vi "Destroy.vi"(8 "error in (no error)":errorcluster, 11 "SolarSystems M266 Old in":refnum<class "SolarSystems M266 Old.lvclass">) -> (3 "SolarSystems M266 Old out":refnum<class "SolarSystems M266 Old.lvclass">)   [LabVIEW 2014, in "SolarSystems M266 Old.lvclass"]
uses:
  SolarSystems M266 Old.lvclass
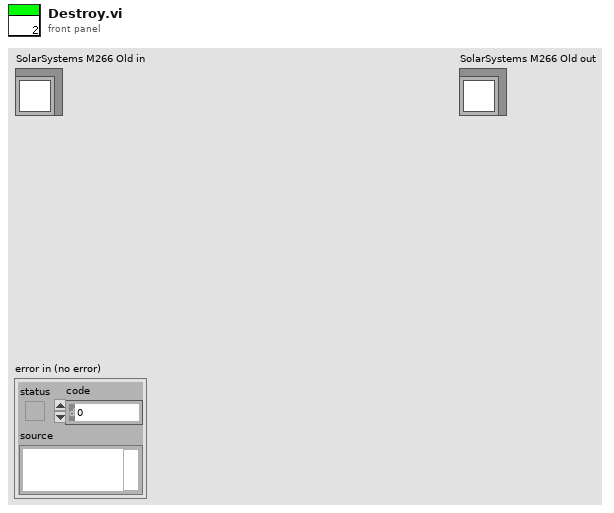
[diagram p1: front panel]
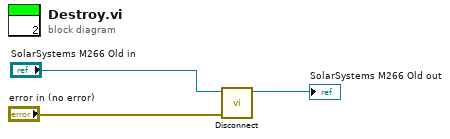
[diagram p0: block diagram]
diagram:
  n1 = call-dynamic "Disconnect.vi"("error in (no error)"="error in (no error)", "SolarSystems M266 Old in"="SolarSystems M266 Old in") -> ("SolarSystems M266 Old out"=→"SolarSystems M266 Old out":refnum<class "SolarSystems M266 Old.lvclass">)  [unwired: 8 in, 1 out]
